vi "FlatToRichni_measurementlink_discovery_v1_ComputeNodeDescriptor.vi"(5 "OutputClusterType":T1, 11 "InputCluster":T2) -> (3 "OutputCluster":T1)   [LabVIEW 2024, in "ni.measurementlink.discovery.v1.api.lvlib"]
uses:
  ni.measurementlink.discovery.v1.api.lvlib
  ni_measurementlink_discovery_v1_ComputeNodeDescriptor_Flat.ctl
  ni_measurementlink_discovery_v1_ComputeNodeDescriptor.ctl
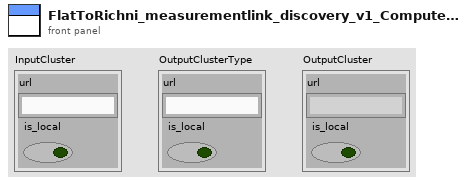
[diagram p1: front panel]
types:
  T1 = typedef "ni.measurementlink.discovery.v1.api.lvlib/ni_measurementlink_discovery_v1_ComputeNodeDescriptor.ctl" = cluster{"url":string, "is_local":bool}
  T2 = typedef "ni.measurementlink.discovery.v1.api.lvlib/ni_measurementlink_discovery_v1_ComputeNodeDescriptor_Flat.ctl" = cluster{"url":string, "is_local":bool}
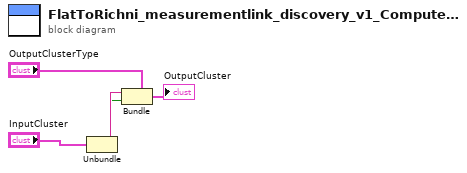
[diagram p0: block diagram]
diagram:
  n1 = Unbundle "Unbundle"("InputCluster") -> ("url"=w2:string, "is_local"=w1:bool)
  n2 = Bundle "Bundle"(cluster="OutputClusterType", "url"=w2, "is_local"=w1) -> (→"OutputCluster":T1)
